vi "Remove Outliers.vi"(1 "Distances (ft)":dbl[](array[numeric])) -> (0 "Mean Distance":dbl)   [LabVIEW 2014]
uses:
  <vilib>/gmath/NI_Gmath.lvlib
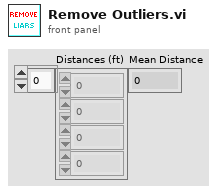
[diagram p1: front panel]
types:
  T1 = enum16{"arithmetic", "geometric", "harmonic", "trimmed", "median"}
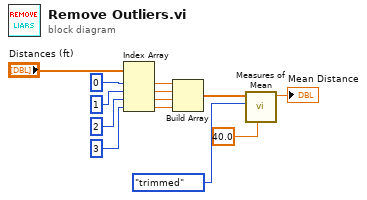
[diagram p0: block diagram]
diagram:
  n1 = Index Array(array="Distances (ft)", index #1=0 ("index"), index #2=1 ("index"), index #3=2 ("index"), index #4=3 ("index")) -> (element #1=w5:dbl, element #2=w4:dbl, element #3=w3:dbl, element #4=w2:dbl)
  n2 = Build Array(w5, w4, w3, w2) -> (w1:dbl[])
  n3 = call <vilib>:"Measures of Mean.vi"("percent (trim)"=40.0, "type"=T1."trimmed", "x array"=w1) -> ("mean value"=→"Mean Distance":dbl)  [unwired: 7 in, 1 out]
